vi "Test State to Error Handler.vi"() -> ()   [LabVIEW 2020]
uses:
  <userlib>/_OpenG.lib/numeric/numeric.llb/Random Number Within Range - I32__ogtk.vi
  <userlib>/_OpenG.lib/error/error.llb/openg_error.lvlib
  <userlib>/_OpenG.lib/numeric/numeric.llb/openg_numeric__ogtk.lvlib
panel:
  out "Error":errorcluster
  out "Error Source Arguments":string
  out "Error Source State":string
  in  "Generate Error":bool
  in  "Stop":bool
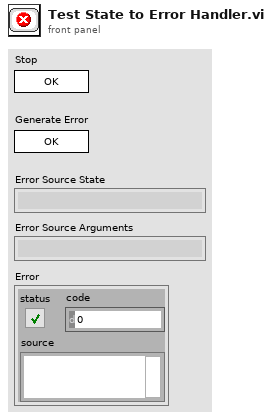
[diagram p1: front panel]
types:
  T1 = enum32{"Invalid", "Standard", "Closed", "Hidden", "Minimized", "Maximized"}
  T2 = enum32{"invalid app kind", "Development System", "Run Time System", "Student Edition", "Embedded LabVIEW", "Evaluation", "Custom"}
  T3 = cluster{"Core":cluster{"Current VI Reference":refnum<vi>, "Close Panel on Exit?":bool}, "Your Boolean data":bool, "Your string data":string}
  T4 = cluster{"Current VI Reference":refnum<vi>, "Close Panel on Exit?":bool}
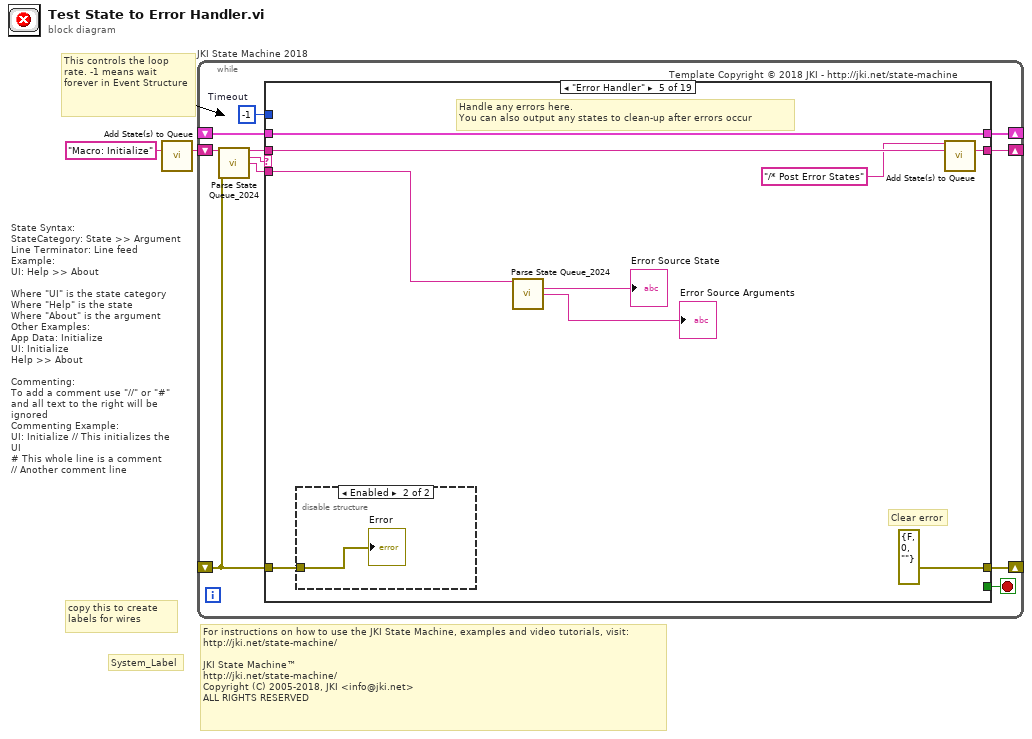
[diagram p0: block diagram]
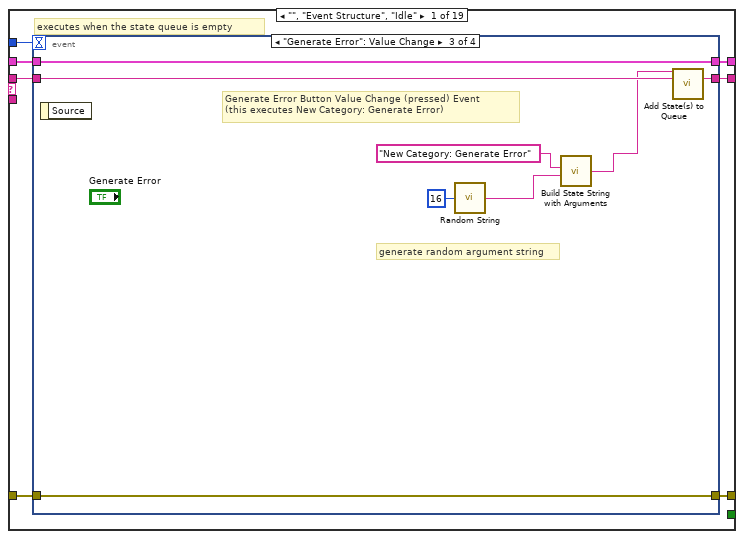
[diagram p2: hidden frame]
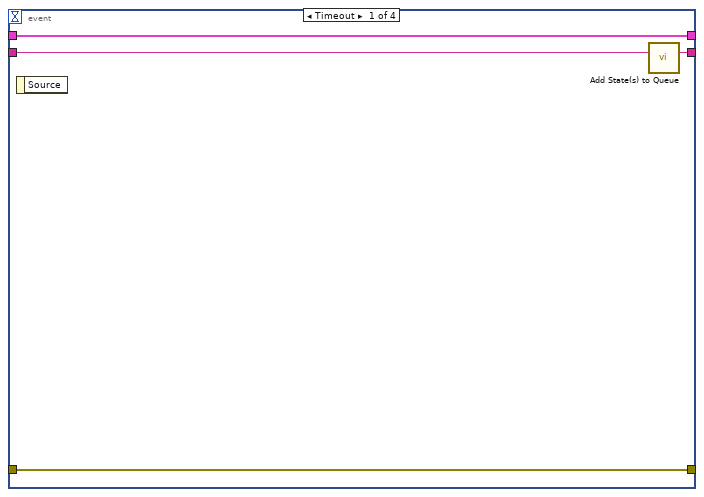
[diagram p3: hidden frame]
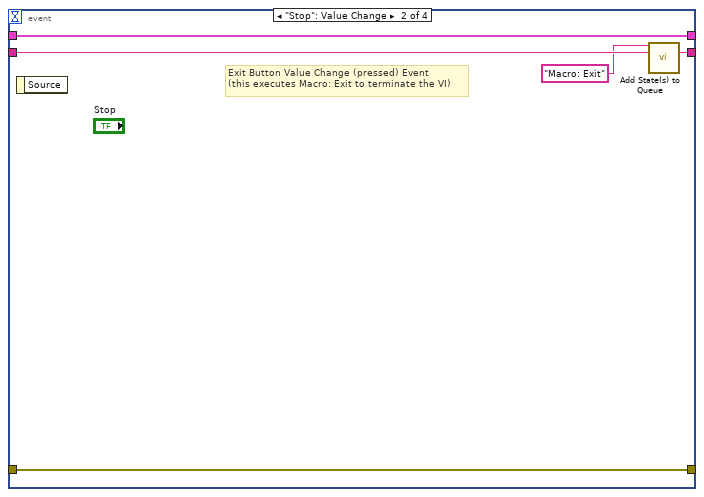
[diagram p4: hidden frame]
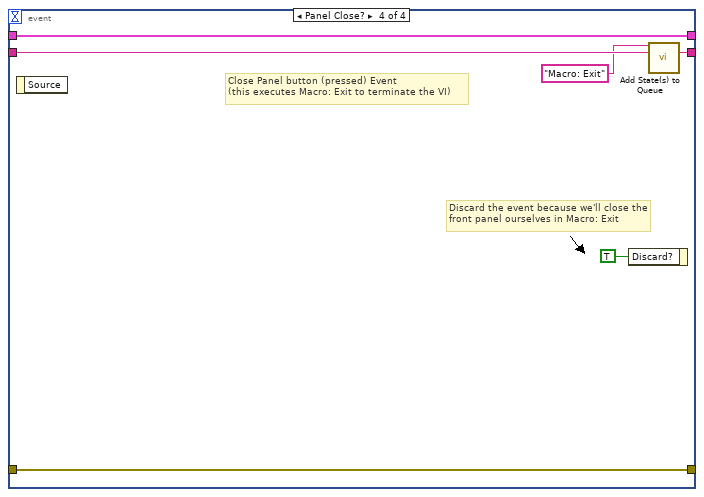
[diagram p5: hidden frame]
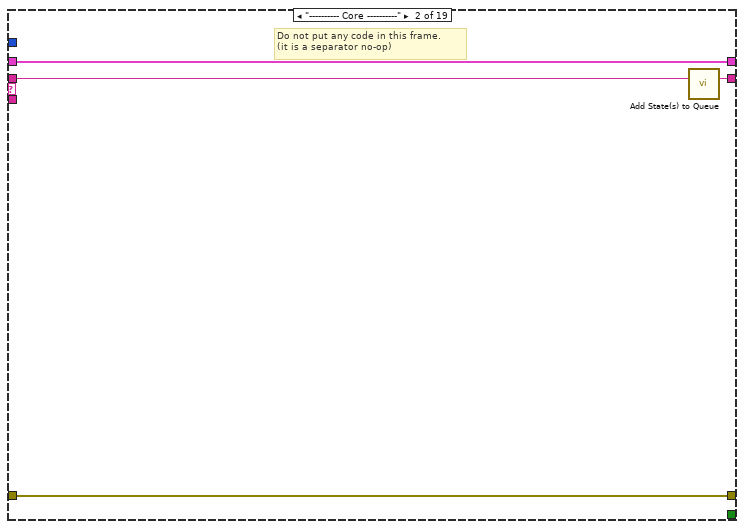
[diagram p6: hidden frame]
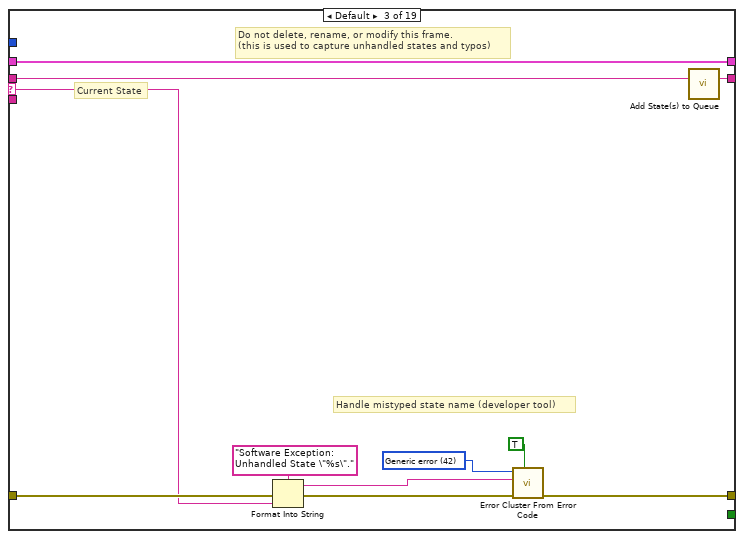
[diagram p7: hidden frame]
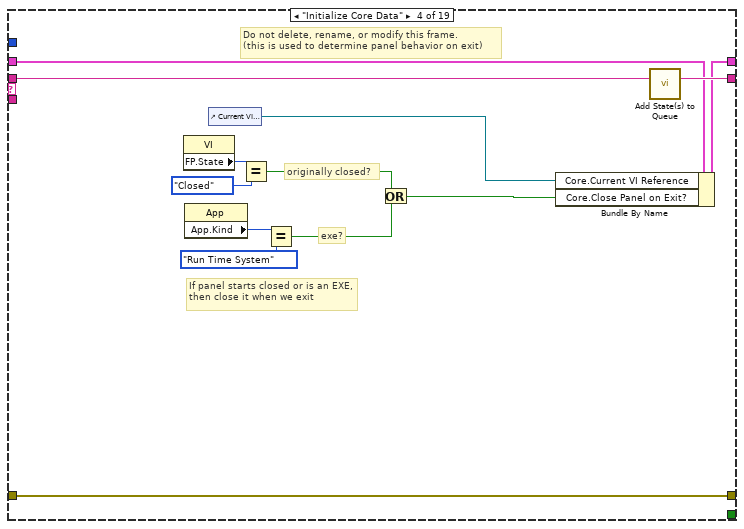
[diagram p8: hidden frame]
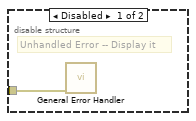
[diagram p9: hidden frame]
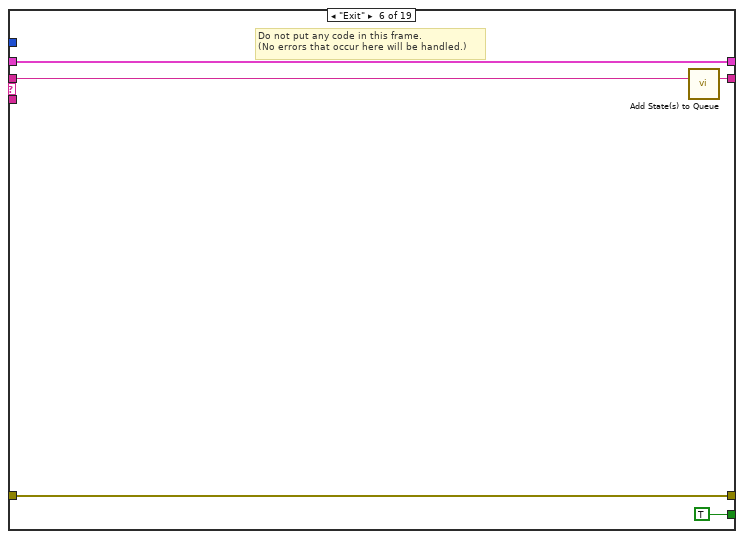
[diagram p10: hidden frame]
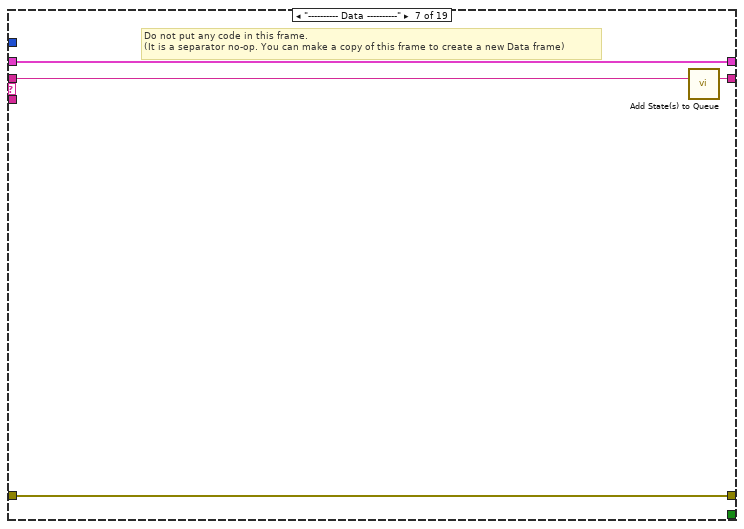
[diagram p11: hidden frame]
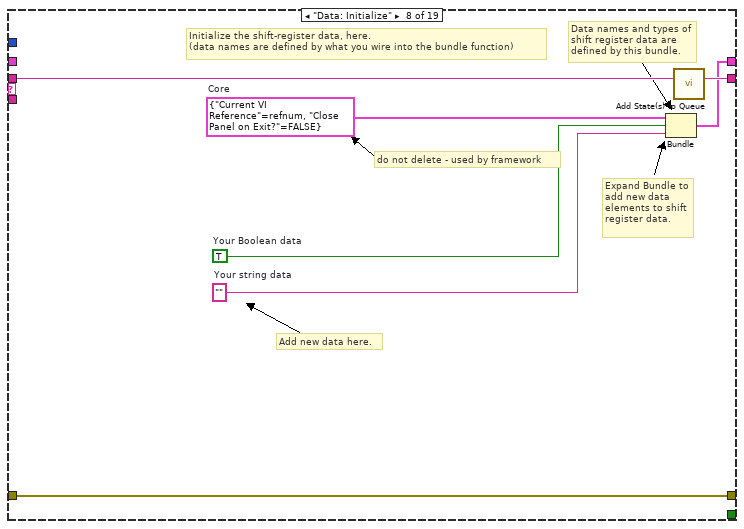
[diagram p12: hidden frame]
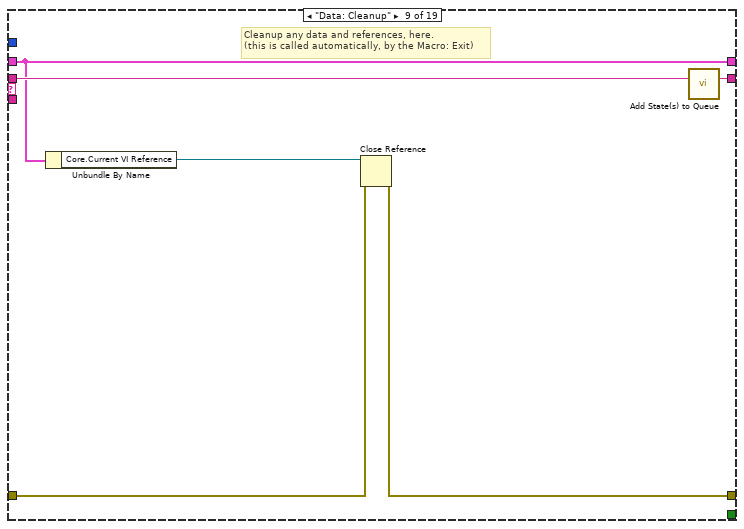
[diagram p13: hidden frame]
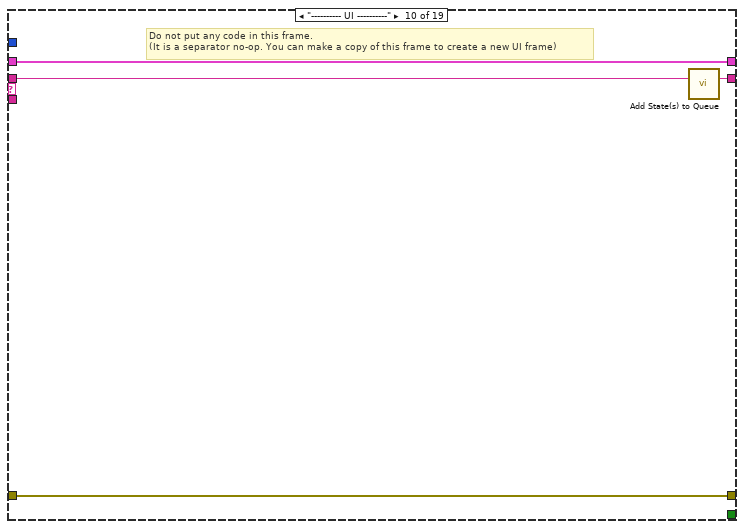
[diagram p14: hidden frame]
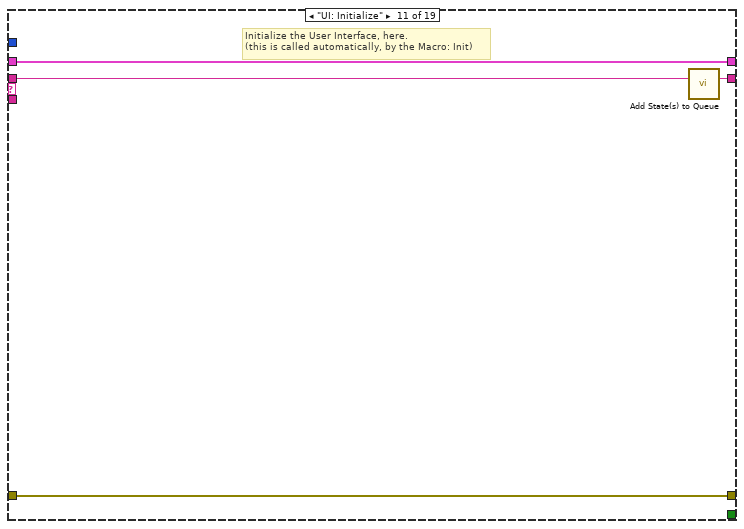
[diagram p15: hidden frame]
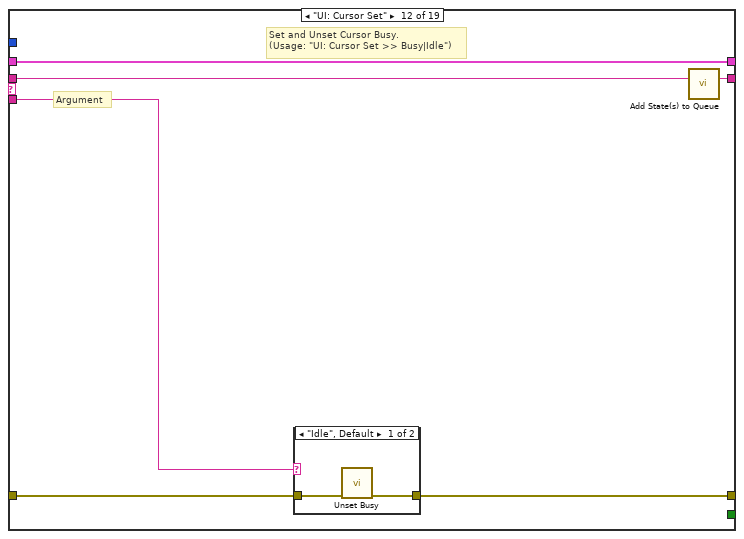
[diagram p16: hidden frame]
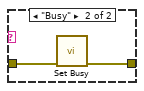
[diagram p17: hidden frame]
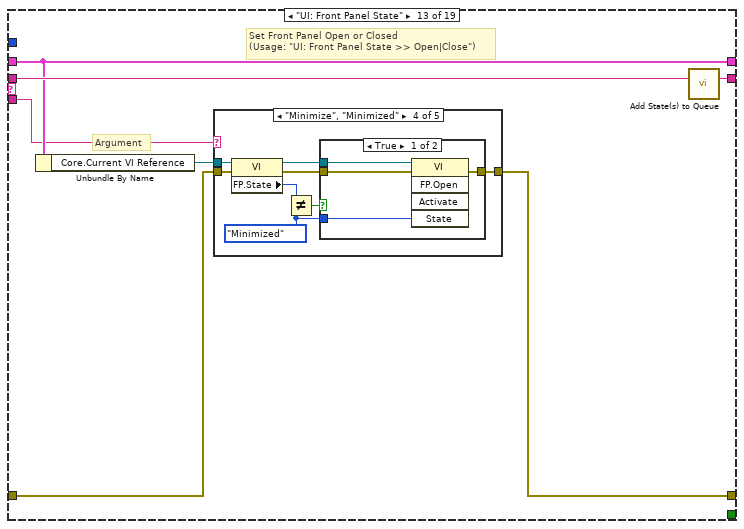
[diagram p18: hidden frame]
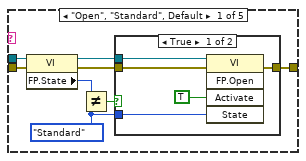
[diagram p19: hidden frame]
diagram:
  # "For instructions on how to use the JKI State Machine, examples and video tutorials, visit:\nhttp://jki.net/state-machine/\n\nJKI State Machine™\nhttp://jki.net/state-machine/\nCopyright (C) 2005-2018, JKI <info@jki.net>\nALL RIGHTS RESERVED"
  # "State Syntax:\nStateCategory: State >> Argument\nLine Terminator: Line feed\nExample:\nUI: Help >> About\n\nWhere \"UI\" is the state category\nWhere \"Help\" is the state\nWhere \"About\" is the argument\nOther Examples:\nApp Data: Initialize\nUI: Initialize\nHelp >> About\n\nCommenting:\nTo add a comment use \"//\" or \"#\" and all text to the right will be ignored\nCommenting Example:\nUI: Initialize // This initializes the UI\n# This whole line is a comment\n// Another comment line"
  # "copy this to create labels for wires"
  # "This controls the loop rate. -1 means wait forever in Event Structure"
  # "System_Label"
  n1 = call "Add State(s) to Queue.vi"("State(s) in (\"\")"="Macro: Initialize") -> ("States Out"=w1:string)  [unwired: 14 in]
  n2 = while "JKI State Machine 2018" {
    shift-right: [w6] -> _
    shift-left: _ -> [w5]
    shift-right: [w9] -> _
    shift-left: _ -> [w3]
    shift-right: [w8] -> _
    shift-left: w1 -> [w10]
    stop <- w7 stop-if-true
    w4 = -1  # Timeout
    # "Template Copyright © 2018 JKI - http://jki.net/state-machine"
    n3 = call "Parse State Queue_2024.vi"("State Queue"=w10, "Error In (no error)"=w3) -> ("Remaining States"=w12:string, "Current State"=w13:string, "Arguments"=w11:string)  [unwired: 11 in]
    n4 = case shown="\"Error Handler\"" w13 {
      selector: w13 -> [_ _ w48 _ _ _ _ _ _ _ _ _ _ _ _ _ _ _ _]
      tunnel: w12 -> [w20 w47 w52 w71 w80 w87 w91 w98 w104 w108 w112 w118 w129 w198 w203 w213 w217 w226 w230]
      tunnel: w11 -> [_ _ _ _ w74 _ _ _ _ _ _ w113 w123 _ _ _ _ _ _]
      tunnel: w5 -> [w18 w44 w50 w64 w77 w85 w88 _ w99 w105 w110 w116 w125 w195 w200 w210 w214 w223 w227]
      tunnel: [w17 w45 w54 w68 errorcluster {"status"=FALSE, "code"=0, "source"=""} ("error out") w84 w89 w95 w100 w106 w109 w114 w126 w196 w201 w211 w215 w222 w228] -> w9
      tunnel: w3 -> [w16 w45 w53 w68 w76 w84 w89 w95 w101 w106 w109 w115 w127 w196 w201 w211 w215 w224 w228]
      tunnel: [w19 w46 w51 w70 w79 w86 w90 w97 w103 w107 w111 w117 w128 w197 w202 w212 w216 w225 w229] -> w8
      tunnel: [_ _ _ _ _ TRUE _ _ _ _ _ _ _ _ _ _ _ _ _] -> w7
      tunnel: [w15 w44 w50 w69 w77 w85 w88 w96 w99 w105 w110 w116 w125 w195 w200 w210 w214 w223 w227] -> w6
      tunnel: w4 -> [w14 _ _ _ _ _ _ _ _ _ _ _ _ _ _ _ _ _ _]
      frame "", "Event Structure", "Idle" {
        # "executes when the state queue is empty"
        n5 = event shown="[2] \"Generate Error\": Value Change" {
          selector: _ -> [_ _ _ _]
          dyn-events: _ -> [_ _ _ _]
          timeout: w14 -> [_ _ _ _]
          tunnel: w20 -> [w24 w29 w37 w43]
          tunnel: [w23 w28 w36 w42] -> w19
          tunnel: w18 -> [w21 w26 w34 w40]
          tunnel: [w22 w27 w35 w41] -> w17
          tunnel: w16 -> [w22 w27 w35 w41]
          tunnel: [w21 w26 w34 w40] -> w15
          event Timeout {
            n6 = event-data() -> ()  [unwired: 1 in, 1 out]
            n7 = call "Add State(s) to Queue.vi"("State(s) in (\"\")"=w24) -> ("States Out"=w23:string)  [unwired: 14 in]
          }
          event "Stop": Value Change {
            # "Exit Button Value Change (pressed) Event\n(this executes Macro: Exit to terminate the VI)"
            n8 = event-data() -> ()  [unwired: 1 in, 1 out]
            n9 = call "Add State(s) to Queue.vi"("State(s) in Front (\"\")"="Macro: Exit", "State(s) in (\"\")"=w29) -> ("States Out"=w28:string)  [unwired: 13 in]
          }
          event "Generate Error": Value Change {
            # "generate random argument string"
            # "Generate Error Button Value Change (pressed) Event\n(this executes New Category: Generate Error)"
            n10 = event-data() -> ()  [unwired: 1 in, 1 out]
            n11 = call "Random String.vi"("Length"=16) -> ("ASCII"=w31:string)  [unwired: 4 in]
            n12 = call "Build State String with Arguments.vi"("Arguments (\"\")"=w31, "State"="New Category: Generate Error") -> ("State with Arguments"=w32:string)  [unwired: 4 in]
            n13 = call "Add State(s) to Queue.vi"("State(s) in Front (\"\")"=w32, "State(s) in (\"\")"=w37) -> ("States Out"=w36:string)  [unwired: 13 in]
          }
          event Panel Close? {
            # "Discard the event because we'll close the front panel ourselves in Macro: Exit"
            # "Close Panel button (pressed) Event\n(this executes Macro: Exit to terminate the VI)"
            n14 = event-data() -> ()  [unwired: 1 in, 1 out]
            n15 = event-data("Discard?"=TRUE) -> ()  [unwired: 1 in, 1 out]
            n16 = call "Add State(s) to Queue.vi"("State(s) in Front (\"\")"="Macro: Exit", "State(s) in (\"\")"=w43) -> ("States Out"=w42:string)  [unwired: 13 in]
          }
        }
      }
      frame "---------- Core ----------" {
        # "Do not put any code in this frame.\n(it is a separator no-op)"
        n17 = call "Add State(s) to Queue.vi"("State(s) in (\"\")"=w47) -> ("States Out"=w46:string)  [unwired: 14 in]
      }
      frame Default {
        w57 = 42 items=["No error", "Argument error", "Memory is full", "Out of zone", "End of file", "File already open", "Generic file I/O error", "File not found", "File permission error", "Disk is full", "Duplicate path", "Too many files open", "System feature not enabled", "Resource file not found", "Cannot add resource", "Resource not found", "Image not found", "Image memory error", "Pen does not exist", "Config type invalid", "Config token not found", "Config parse error", "Config memory error", "Bad external code format", "Bad external code offset", "External code not present", "Null window", "Destroy window error", "Null menu", "Print aborted", "Bad print record", "Print driver error", "Windows error during printing", "Memory error during printing", "Print dialog error", "Generic print error", "Invalid device refnum", "Device not found", "Device parameter error", "Device unit error", "Cannot open device", "Device call aborted", "Generic error", "Cancelled by user", "Object ID too low", "Object ID too high", "Object not in heap", "Unknown heap", "Unknown object (invalid DefProc)", "Unknown object (DefProc not in table)", "Message out of range", "Invalid (null) method", "Unknown message", "Manager call not supported", "Bad address", "Network operation in progress", "Network operation timed out", "Connection is busy", "Network attribute not supported", "Network error", "Address in use", "System out of memory", "Connection aborted", "Connection refused", "Not connected", "Already connected", "Connection closed", "Initialization error (interapplication manager)", "Bad occurrence", "Wait on unbound occurrence handler", "Occurrence queue overflow", "Datalog type conflict", "Unused", "Unrecognized type (interapplication manager)", "Memory corrupt", "Failed to make temporary DLL", "Old CIN version", "Drag socket not found", "Failed to load drop-object", "Failed to register OLE object", "Failed to release OLE object", "Format specifier type mismatch", "Unknown format specifier", "Too few format specifiers", "Too many format specifiers", "Scan failed", "Newer CIN version", "Error converting to variant", "Runtime menu error", "Password tampered", "Variant attribute not found", "Incompatible variant data type", "Event data is not available", "Event Store is not present", "Occurrence is not found", "Event Queue is not created", "Event info is not available", "Refnum passed is NULL", "Error retrieving Class GUID", "Error retrieving CoClass GUID", "Error retrieving TypeLib GUID.", "Bad built application magic bytes.", "Specific driver is different from the specific driver associated with the Logical Name.", "There is no session opened to the class driver.", "Max Error", "MAX - Error with config objects", "MAX - Error loading configuration", "MAX - Group not supported"]
        # "Current State"
        # "Do not delete, rename, or modify this frame.\n(this is used to capture unhandled states and typos)"
        # "Handle mistyped state name (developer tool)"
        n18 = Format Into String(format string="Software Exception: Unhandled State \"%s\"." ("message"), error in=w53, w48) -> (resulting string=w56:string, error out=w55:errorcluster)  [unwired: 1 in]
        n19 = call <vilib>:"Error Cluster From Error Code.vi"("show call chain? (False)"=TRUE, "error in (no error)"=w55, "error message (\"\")"=w56, "error code (0)"=w57) -> ("error out"=w54:errorcluster)  [unwired: 5 in]
        n20 = call "Add State(s) to Queue.vi"("State(s) in (\"\")"=w52) -> ("States Out"=w51:string)  [unwired: 14 in]
      }
      frame "Initialize Core Data" {
        # "Do not delete, rename, or modify this frame.\n(this is used to determine panel behavior on exit)"
        # "originally closed?"
        # "exe?"
        # "If panel starts closed or is an EXE, then close it when we exit"
        n21 = property class="VI"() -> ("FP.State"=w61:T1)  [unwired: 2 in, 2 out]
        n22 = property class="App"() -> ("App.Kind"=w67:T2)  [unwired: 2 in, 2 out]
        n23 = control-ref of="Current VI Reference"() -> (w62:refnum<vi>)
        n24 = Equal?(x=w61, y=T1."Closed" ("Front Panel Window:State")) -> (x = y?=w59:bool)
        n25 = Equal?(x=w67, y=T2."Run Time System" ("Application:Kind")) -> (x = y?=w65:bool)
        n26 = Or(x=w59, y=w65) -> (x .or. y?=w63:bool)
        n27 = Bundle By Name(cluster=w64, "Core.Current VI Reference"=w62, "Core.Close Panel on Exit?"=w63) -> (w69:T3)
        n28 = call "Add State(s) to Queue.vi"("State(s) in (\"\")"=w71) -> ("States Out"=w70:string)  [unwired: 14 in]
      }
      frame "Error Handler" {
        # "Handle any errors here.\nYou can also output any states to clean-up after errors occur"
        # "Clear error"
        n29 = disable-structure shown="Enabled" {
          disable-tunnel: w76 -> [w81 w82]
          frame Disabled {
            # "Unhandled Error -- Display it"
            n30 = call <vilib>:"General Error Handler.vi"("error in (no error)"=w81) -> ()  [unwired: 10 in, 5 out]
          }
          frame Enabled {
            "Error" <- w82
          }
        }
        n31 = call "Parse State Queue_2024.vi"("State Queue"=w74) -> ("Current State"=→"Error Source State":string, "Arguments"=→"Error Source Arguments":string)  [unwired: 12 in, 1 out]
        n32 = call "Add State(s) to Queue.vi"("State(s) in Front (\"\")"="/* Post Error States", "State(s) in (\"\")"=w80) -> ("States Out"=w79:string)  [unwired: 13 in]
      }
      frame "Exit" {
        # "Do not put any code in this frame.\n(No errors that occur here will be handled.)"
        n33 = call "Add State(s) to Queue.vi"("State(s) in (\"\")"=w87) -> ("States Out"=w86:string)  [unwired: 14 in]
      }
      frame "---------- Data ----------" {
        # "Do not put any code in this frame.\n(It is a separator no-op. You can make a copy of this frame to create a new Data frame)"
        n34 = call "Add State(s) to Queue.vi"("State(s) in (\"\")"=w91) -> ("States Out"=w90:string)  [unwired: 14 in]
      }
      frame "Data: Initialize" {
        w92 = T4 {"Current VI Reference"=refnum, "Close Panel on Exit?"=FALSE}  # Core
        w94 = TRUE  # Your Boolean data
        w93 = ""  # Your string data
        # "do not delete - used by framework"
        # "Expand Bundle to add new data elements to shift register data."
        # "Add new data here."
        # "Data names and types of shift register data are defined by this bundle."
        # "Initialize the shift-register data, here.\n(data names are defined by what you wire into the bundle function)"
        n35 = Bundle("Core"=w92, "Your Boolean data"=w94, "Your string data"=w93) -> (w96:T3)  [unwired: 1 in]
        n36 = call "Add State(s) to Queue.vi"("State(s) in (\"\")"=w98) -> ("States Out"=w97:string)  [unwired: 14 in]
      }
      frame "Data: Cleanup" {
        # "Cleanup any data and references, here.\n(this is called automatically, by the Macro: Exit)"
        n37 = Unbundle By Name(w99) -> ("Core.Current VI Reference"=w102:refnum<vi>)
        n38 = Close Reference(reference=w102, error in (no error)=w101) -> (error out=w100:errorcluster)
        n39 = call "Add State(s) to Queue.vi"("State(s) in (\"\")"=w104) -> ("States Out"=w103:string)  [unwired: 14 in]
      }
      frame "---------- UI ----------" {
        # "Do not put any code in this frame.\n(It is a separator no-op. You can make a copy of this frame to create a new UI frame)"
        n40 = call "Add State(s) to Queue.vi"("State(s) in (\"\")"=w108) -> ("States Out"=w107:string)  [unwired: 14 in]
      }
      frame "UI: Initialize" {
        # "Initialize the User Interface, here.\n(this is called automatically, by the Macro: Init)"
        n41 = call "Add State(s) to Queue.vi"("State(s) in (\"\")"=w112) -> ("States Out"=w111:string)  [unwired: 14 in]
      }
      frame "UI: Cursor Set" {
        # "Argument"
        # "Set and Unset Cursor Busy.\n(Usage: \"UI: Cursor Set >> Busy|Idle\")"
        n42 = case shown="\"Idle\", Default" w113 {
          tunnel: w115 -> [w120 w122]
          tunnel: [w119 w121] -> w114
          frame "Idle", Default {
            n43 = call <vilib>:"Unset Busy.vi"("error in (no error)"=w120) -> ("error out"=w119:errorcluster)  [unwired: 10 in]
          }
          frame "Busy" {
            n44 = call <vilib>:"Set Busy.vi"("error in (no error)"=w122) -> ("error out"=w121:errorcluster)  [unwired: 9 in, 1 out]
          }
        }
        n45 = call "Add State(s) to Queue.vi"("State(s) in (\"\")"=w118) -> ("States Out"=w117:string)  [unwired: 14 in]
      }
      frame "UI: Front Panel State" {
        # "Argument"
        # "Set Front Panel Open or Closed\n(Usage: \"UI: Front Panel State >> Open|Close\")"
        n46 = Unbundle By Name(w125) -> ("Core.Current VI Reference"=w124:refnum<vi>)
        n47 = case shown="\"Minimize\", \"Minimized\"" w123 {
          tunnel: w127 -> [w135 w150 w161 w174 w187]
          tunnel: [w137 w151 w163 w176 w189] -> w126
          tunnel: w124 -> [w136 w148 w162 w175 w188]
          frame "Open", "Standard", Default {
            w130 = T1."Standard" ("State")
            n48 = property class="VI"(reference=w136, error in=w135) -> (reference out=w133:refnum<vi>, error out=w134:errorcluster, "FP.State"=w132:T1)
            n49 = Not Equal?(x=w132, y=w130) -> (x != y?=w131:bool)
            n50 = case shown="True" w131 {
              tunnel: [w141 w143] -> w137
              tunnel: w134 -> [w140 w143]
              tunnel: w133 -> [w139 _]
              tunnel: w130 -> [w138 _]
              frame True {
                n51 = invoke class="VI" method="FP.Open"(reference=w139, error in=w140, "Activate"=TRUE, "State"=w138) -> (error out=w141:errorcluster)  [unwired: 1 in, 4 out]
              }
              frame False {
              }
            }
          }
          frame "Close", "Closed" {
            n52 = property class="VI"(reference=w148, error in=w150) -> (reference out=w147:refnum<vi>, error out=w149:errorcluster, "FP.State"=w145:T1)
            n53 = Not Equal?(x=w145, y=T1."Closed" ("Front Panel Window:State")) -> (x != y?=w144:bool)
            n54 = case shown="True" w144 {
              tunnel: [w152 w155] -> w151
              tunnel: w149 -> [w152 w154]
              tunnel: w147 -> [_ w153]
              frame False {
              }
              frame True {
                n55 = invoke class="VI" method="FP.Close"(reference=w153, error in=w154) -> (error out=w155:errorcluster)  [unwired: 1 in, 2 out]
              }
            }
          }
          frame "Hidden", "Hide" {
            w156 = T1."Hidden" ("State")
            n56 = property class="VI"(reference=w162, error in=w161) -> (reference out=w159:refnum<vi>, error out=w160:errorcluster, "FP.State"=w158:T1)
            n57 = Not Equal?(x=w158, y=w156) -> (x != y?=w157:bool)
            n58 = case shown="True" w157 {
              tunnel: [w167 w168] -> w163
              tunnel: w160 -> [w166 w168]
              tunnel: w159 -> [w165 _]
              tunnel: w156 -> [w164 _]
              frame True {
                n59 = invoke class="VI" method="FP.Open"(reference=w165, error in=w166, "State"=w164) -> (error out=w167:errorcluster)  [unwired: 2 in, 4 out]
              }
              frame False {
              }
            }
          }
          frame "Minimize", "Minimized" {
            w169 = T1."Minimized" ("State")
            n60 = property class="VI"(reference=w175, error in=w174) -> (reference out=w172:refnum<vi>, error out=w173:errorcluster, "FP.State"=w171:T1)
            n61 = Not Equal?(x=w171, y=w169) -> (x != y?=w170:bool)
            n62 = case shown="True" w170 {
              tunnel: [w180 w181] -> w176
              tunnel: w173 -> [w179 w181]
              tunnel: w172 -> [w178 _]
              tunnel: w169 -> [w177 _]
              frame True {
                n63 = invoke class="VI" method="FP.Open"(reference=w178, error in=w179, "State"=w177) -> (error out=w180:errorcluster)  [unwired: 2 in, 4 out]
              }
              frame False {
              }
            }
          }
          frame "Maximize", "Maximized" {
            w182 = T1."Maximized" ("State")
            n64 = property class="VI"(reference=w188, error in=w187) -> (reference out=w185:refnum<vi>, error out=w186:errorcluster, "FP.State"=w184:T1)
            n65 = Not Equal?(x=w184, y=w182) -> (x != y?=w183:bool)
            n66 = case shown="True" w183 {
              tunnel: [w193 w194] -> w189
              tunnel: w186 -> [w192 w194]
              tunnel: w185 -> [w191 _]
              tunnel: w182 -> [w190 _]
              frame True {
                n67 = invoke class="VI" method="FP.Open"(reference=w191, error in=w192, "State"=w190) -> (error out=w193:errorcluster)  [unwired: 2 in, 4 out]
              }
              frame False {
              }
            }
          }
        }
        n68 = call "Add State(s) to Queue.vi"("State(s) in (\"\")"=w129) -> ("States Out"=w128:string)  [unwired: 14 in]
      }
      frame "---------- Macro ----------" {
        # "Do not put any code in this frame.\n(It is a separator no-op. You can make a copy of this frame to create a new Macro frame)"
        n69 = call "Add State(s) to Queue.vi"("State(s) in (\"\")"=w198) -> ("States Out"=w197:string)  [unwired: 14 in]
      }
      frame "Macro: Initialize" {
        w199 = "Data: Initialize\nInitialize Core Data\nUI: Initialize\nUI: Front Panel State >> Open"  # Data: Initialize Initialize Core Data UI: Initialize UI: Front Panel State >> Open
        # "Initialization Macro\n(This is called once, when the VI starts)"
        n70 = call "Add State(s) to Queue.vi"("State(s) in Front (\"\")"=w199, "State(s) in (\"\")"=w203) -> ("States Out"=w202:string)  [unwired: 13 in]
      }
      frame "Macro: Exit" {
        # "Exit Macro\n(This is called once, when the VI exits)"
        n71 = Unbundle By Name(w210) -> ("Core.Close Panel on Exit?"=w209:bool)
        n72 = Select(t="UI: Front Panel State >> Close", s=w209, f="") -> (s? t:f=w206:string)
        n73 = call "Add State(s) to Queue.vi"("State(s) in (\"\")"=w206, "State(s) at Back (\"\")"="Data: Cleanup\nExit") -> ("States Out"=w204:string)  [unwired: 13 in]
        n74 = call "Add State(s) to Queue.vi"("State(s) in Front (\"\")"=w204, "State(s) in (\"\")"=w213) -> ("States Out"=w212:string)  [unwired: 13 in]
      }
      frame "---------- New Category ----------" {
        # "Template Separator\n(You can make a copy of, or modify, this frame)"
        n75 = call "Add State(s) to Queue.vi"("State(s) in (\"\")"=w217) -> ("States Out"=w216:string)  [unwired: 14 in]
      }
      frame "New Category: Generate Error" {
        # "Your code here.\n(You can make a copy of, or modify, this frame)"
        n76 = call-poly <userlib>:"Random Number Within Range__ogtk.vi"("High"=-9999 ("code"), "Low"=-999) -> ("Random Number"=w218:i32)  [unwired: 3 in]
        n77 = call <userlib>:"Build Error Cluster__ogtk.vi"("code"=w218) -> ("error out"=w221:errorcluster)  [unwired: 1 in]
        n78 = Merge Errors(w221, w224) -> (w222:errorcluster)
        n79 = call "Add State(s) to Queue.vi"("State(s) in (\"\")"=w226) -> ("States Out"=w225:string)  [unwired: 14 in]
      }
      frame "New Category: 2" {
        # "Your code here.\n(You can make a copy of, or modify, this frame)"
        n80 = call "Add State(s) to Queue.vi"("State(s) in (\"\")"=w230) -> ("States Out"=w229:string)  [unwired: 14 in]
      }
    }
  }
